vi "IMAQ FPGA FIFO to Pixel Bus U8x1.vi"(6 "Ready For Output":bool=TRUE, 10 "Image Size":T2, 11 "Source Image FIFO":refnum<k21>) -> (0 "Output Valid":bool, 2 "Source FIFO Status":T1, 3 "Pixel Bus Out":T3)   [LabVIEW 2017, in "NI_VDM_FPGA_Basics.lvlib"]
doc: "Reads image pixels out of the specified FIFO and returns a Pixel Bus cluster of the requested type. The Pixel Bus contains the pixel data from the FIFO along with some additional flags that indicate when the pixel data is valid, an end of a line has been reached, or an end of the image has been reached. The Pixel Bus is used to pass image data to all of the other VIs in the NI Vision Development Module for FPGA library. Only one of the DV, EOL, and EOI flags in the Pixel Bus cluster will assert on a given clock cycle. When the last pixel of an image is reached, the Pixel Bus will contain the pixel data and the DV flag will be TRUE and the EOL and EOI flags will be FALSE. The next clock cycle, the EOL flag will be TRUE and the DV and EOI flags will be FALSE. The following clock cycle, the EOI flag will be TRUE and the DV and EOL flags will be FALSE."
uses:
  <vilib>/visionFPGA/NI_VDM_FPGA_Basics.lvlib
  <vilib>/rvi/DataTransferAndStorage/Container/XNode/niFpgaContainer.xnode
  <vilib>/rvi/FIFO/Fifo_Resource/niFpgaFifoEmulationRefIn.vi
  <vilib>/visionFPGA/Controls/IMAQ FPGA Pixel Bus u8x1.ctl
  <vilib>/visionFPGA/Controls/IMAQ FPGA Source FIFO Status.ctl
  <vilib>/visionFPGA/Controls/IMAQ FPGA Image Size.ctl
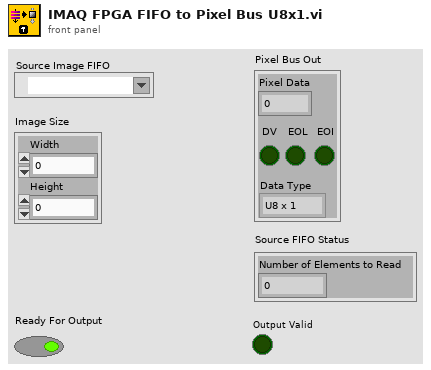
[diagram p1: front panel]
types:
  T1 = typedef "IMAQ FPGA Source FIFO Status.ctl" = cluster{"Number of Elements to Read":u32}
  T2 = typedef "IMAQ FPGA Image Size.ctl" = cluster{"Width":u32, "Height":u32}
  T3 = typedef "IMAQ FPGA Pixel Bus u8x1.ctl" = cluster{"Pixel Data":u8, "DV":bool, "EOL":bool, "EOI":bool, "Data Type":enum16{"U8 x 1"}}
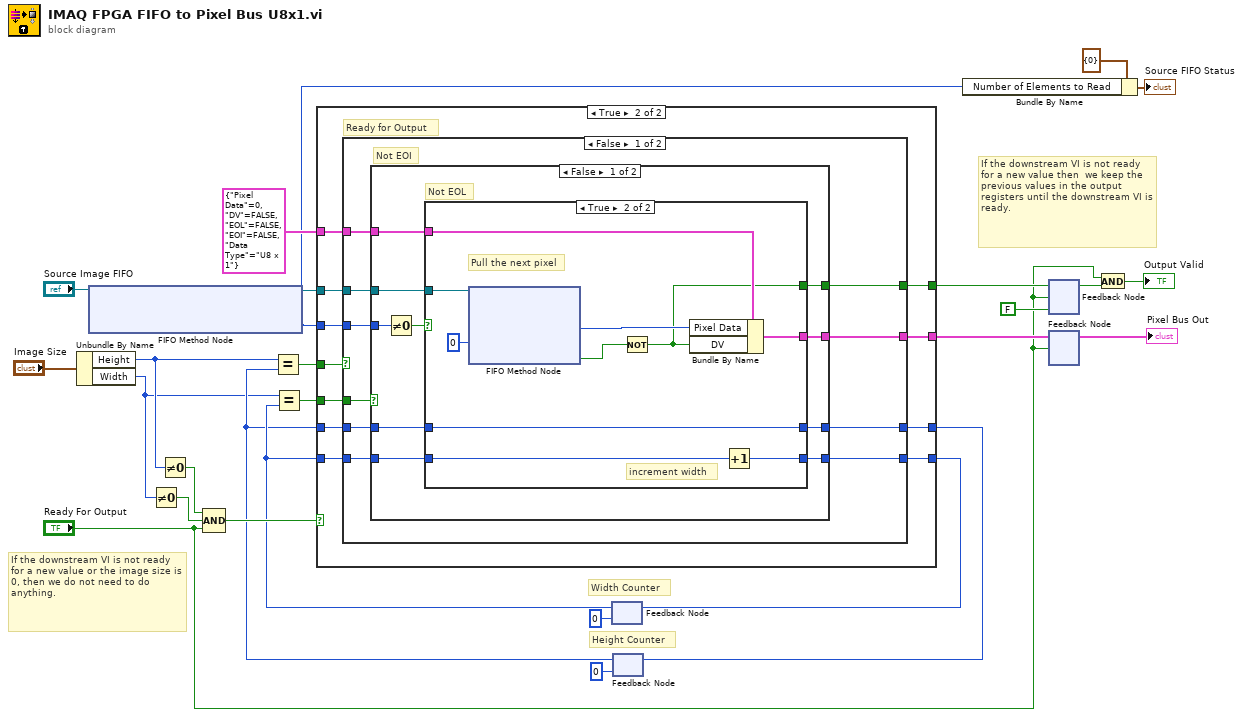
[diagram p0: block diagram]
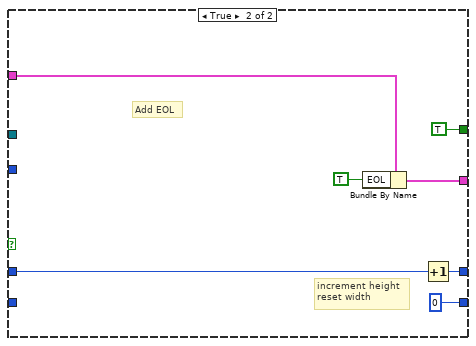
[diagram p4: hidden frame]
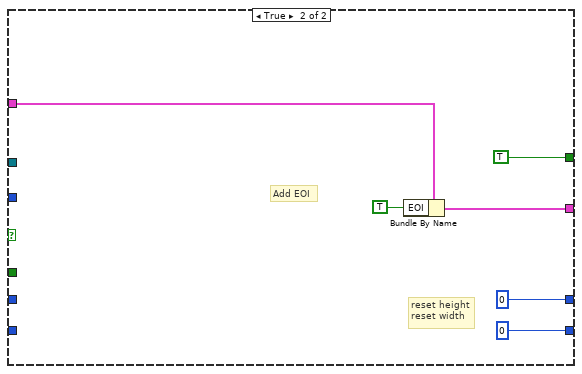
[diagram p5: hidden frame]
diagram:
  # "If the downstream VI is not ready for a new value then  we keep the previous values in the output registers until the downstream VI is ready."
  # "If the downstream VI is not ready for a new value or the image size is 0, then we do not need to do anything."
  # "Height Counter"
  # "Width Counter"
  n1 = Unbundle By Name("Image Size") -> ("Height"=w10:u32, "Width"=w9:u32)
  n2 = xnode ("FIFO Method Node")("FIFO In"="Source Image FIFO") -> ("Number of Elements to Read"=w1:u32, "FIFO Out"=w17:refnum<k21>)
  n3 = Not Equal To 0?(x=w9) -> (x != 0?=w15:bool)
  n4 = Not Equal To 0?(x=w10) -> (x != 0?=w14:bool)
  n5 = Compound Arithmetic op=AND(w14, w15, "Ready For Output") -> (w16:bool)
  n6 = feedback #1(u32 0 ("Image Width")) -> (w13:u32)
  n7 = Equal?(x=w9, y=w13) -> (x = y?=w24:bool)
  n8 = feedback #2(u32 0 ("Image Width")) -> (w12:u32)
  n9 = Equal?(x=w10, y=w12) -> (x = y?=w26:bool)
  n10 = case shown="True" w16 {
    tunnel: w26 -> [_ w40]
    tunnel: T3 {"Pixel Data"=0, "DV"=FALSE, "EOL"=FALSE, "EOI"=FALSE, "Data Type"=enum."U8 x 1"} ("Pixel Bus Out") -> [_ w39]
    tunnel: w24 -> [_ w38]
    tunnel: w1 -> [_ w37]
    tunnel: [_ w36] -> w23
    tunnel: [w28 w35] -> w21
    tunnel: w13 -> [w28 w34]
    tunnel: [w29 w33] -> w19
    tunnel: w12 -> [w29 w32]
    tunnel: [_ w31] -> w18
    tunnel: w17 -> [_ w30]
    frame False {
      # "Do nothing...\nDown stream VI is not ready for new data."
    }
    frame True {
      # "Ready for Output"
      n11 = case shown="False" w40 {
        tunnel: w38 -> [w50 _]
        tunnel: [w49 TRUE ("EOI")] -> w36
        tunnel: [w48 w81] -> w31
        tunnel: w32 -> [w47 _]
        tunnel: w34 -> [w46 _]
        tunnel: [w45 u16 0 ("Height Counter")] -> w33
        tunnel: [w44 u16 0 ("Width Counter")] -> w35
        tunnel: w37 -> [w43 _]
        tunnel: w39 -> [w42 w80]
        tunnel: w30 -> [w41 _]
        frame False {
          # "Not EOI"
          n12 = case shown="False" w50 {
            tunnel: [w58 w78] -> w48
            tunnel: [w57 TRUE ("EOI")] -> w49
            tunnel: w47 -> [w56 w76]
            tunnel: w46 -> [w55 _]
            tunnel: [w53 w74] -> w45
            tunnel: [w54 u16 0 ("Width Counter")] -> w44
            tunnel: w43 -> [w59 _]
            tunnel: w42 -> [w52 w73]
            tunnel: w41 -> [w51 _]
            frame False {
              # "Not EOL"
              n13 = Not Equal To 0?(x=w59) -> (x != 0?=w60:bool)
              n14 = case shown="True" w60 {
                tunnel: [_ w71] -> w58
                tunnel: [_ w63] -> w57
                tunnel: w56 -> [w61 w68]
                tunnel: w55 -> [w62 w70]
                tunnel: [w62 w69] -> w54
                tunnel: [w61 w68] -> w53
                tunnel: w52 -> [_ w66]
                tunnel: w51 -> [_ w65]
                frame False {
                  # "Do nothing...\nnot EOI, not EOL, \nand no DMA data available"
                }
                frame True {
                  # "increment width"
                  # "Pull the next pixel"
                  n15 = xnode ("FIFO Method Node")("Timeout"=0, "FIFO In"=w65) -> ("Element"=w67:u8, "Timed Out?"=w64:bool)  [unwired: 1 out]
                  n16 = Not(x=w64) -> (.not. x?=w63:bool)
                  n17 = Bundle By Name(cluster=w66, "Pixel Data"=w67, "DV"=w63) -> (w71:T3)
                  n18 = Increment(x=w70) -> (x+1=w69:u32)
                }
              }
            }
            frame True {
              # "increment height\nreset width"
              # "Add EOL"
              n19 = Bundle By Name(cluster=w73, "EOL"=TRUE) -> (w78:T3)
              n20 = Increment(x=w76) -> (x+1=w74:u32)
            }
          }
        }
        frame True {
          # "reset height\nreset width"
          # "Add EOI"
          n21 = Bundle By Name(cluster=w80, "EOI"=TRUE) -> (w81:T3)
        }
      }
    }
  }
  n22 = feedback-in #1(w21) -> ()
  n23 = feedback-in #2(w19) -> ()
  n24 = Bundle By Name(cluster=T1 {"Number of Elements to Read"=0} ("FIFO Status"), "Number of Elements to Read"=w1) -> (→"Source FIFO Status":T1)
  n25 = feedback-in #3(w23, "Ready For Output") -> ()
  n26 = feedback #3(FALSE ("EOI")) -> (w8:bool)
  n27 = feedback-in #4(w18, "Ready For Output") -> ()
  n28 = feedback #4() -> (→"Pixel Bus Out":T3)  [unwired: 1 in]
  n29 = And(x="Ready For Output", y=w8) -> (x .and. y?=→"Output Valid":bool)
